vi "RS-xxx Factory.vi"(8 "error in (no error)":errorcluster, 10 "RS-xxx settings":T1) -> (0 "error out":errorcluster, 3 "RS-xxx out":refnum<class "RS-xxx.lvclass">)   [LabVIEW 2018, in "Protocols.lvlib" / "RS-xxx.lvclass"]
doc: "Instantiate an RS-xxx Protocol Object using the provided RS-xxx Port Settings\n\nInput: \nPort: specifies the resource to be opened.\nBaud Rate: is the rate of transmission.\nData Bits: is the number of bits in the incoming data.The value of data bits is between five and eight.\nParity: specifies the parity used for every frame to be transmitted or received. This input accepts the following values. \n\n 0 - no parity (default) \n 1 - odd parity \n 2 - even parity \n 3 - mark parity \n 4 - space parity\n\nFlow Control: sets the type of control used by the transfer mechanism. This input accepts the following values.\n\n 0 - None (default)—The transfer mechanism does not use flow control. Buffers on both sides of the connection are assumed to be large enough to hold all data transferred. \n 1 - XON/XOFF—The transfer mechanism uses the XON and XOFF characters to perform flow control. The transfer mechanism controls input flow by sending XOFF when the receive buffer is nearly full, and it controls the output flow by suspending transmission when XOFF is received. \n 2 - RTS/CTS—The transfer mechanism uses the RTS output signal and the CTS input signal to perform flow control. The transfer mechanism controls input flow by unasserting the RTS signal when the receive buffer is nearly full, and it controls output flow by suspending the transmission when the CTS signal is unasserted. \n 3 - XON/XOFF and RTS/CTS—The transfer mechanism uses the XON and XOFF characters and the RTS output signal and CTS input signal to perform flow control. The transfer mechanism controls input flow by sending XOFF and unasserting the RTS signal when the receive buffer is nearly full, and it controls the output flow by suspending transmission when XOFF is received and the CTS is unasserted. \n 4 - DTR/DSR—The transfer mechanism uses the DTR output signal and the DSR input signal to perform flow control. The transfer mechanism controls input flow by unasserting the DTR signal when the receive buffer is nearly full, and it controls output flow by suspending the transmission when the DSR signal is unasserted. \n 5 - XON/XOFF and DTR/DSR—The transfer mechanism uses the XON and XOFF characters and the DTR output signal and DSR input signal to perform flow control. The transfer mechanism controls input flow by sending XOFF and unasserting the DTR signal when the receive buffer is nearly full, and it controls the output flow by suspending transmission when XOFF is received and the DSR signal is unasserted. \n\nXON: specifies the XON character\nXOFF: specifies the XOFF character\nEnd Read on Termination Character: ends reading the transfered data when encountering the specified termination character\nEnd Write on Termination Character: ends writing the message when encountering the specified termination character\n\nOutput:\n\nRS-xxx Out: RS-xxx object created using the provided RS-xxx Settings"
uses:
  RS-xxx.lvclass
  RS-xxx Settings.ctl
  RS-xxx.lvclass/RS-xxx.ctl
  Data Access/Write PortSettings.vi
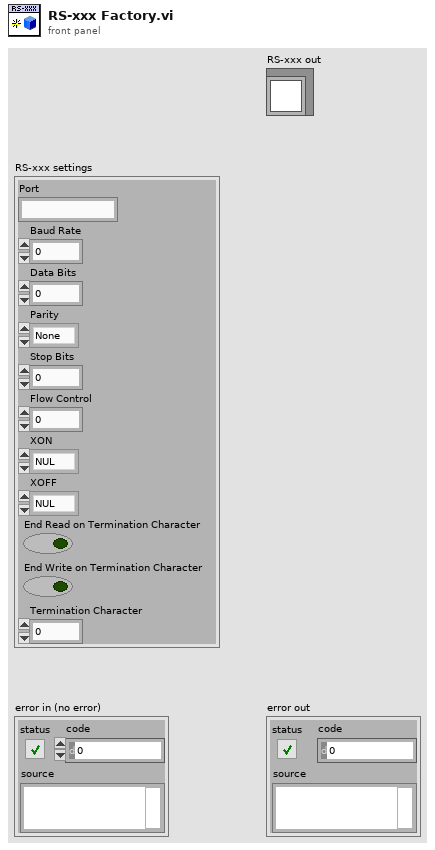
[diagram p1: front panel]
types:
  T1 = typedef "Protocols.lvlib/RS-xxx.lvclass/RS-xxx Settings.ctl" = cluster{"Port":string, "Baud Rate":u32, "Data Bits":u16, "Parity":enum16{"None", "Odd", "Even", "Mark", "Space"}, "Stop Bits":u16, "Flow Control":u16, "XON":enum16{"NUL", "SOH", "STX", "ETX", "EOT", "ENQ", "ACK", "BEL", "BS", "HT", "LF", "VT", "FF", "CR", "SO", "SI", "DLE", "DC1", "DC2", "DC3", "DC4", "NAK", "SYN", "ETB", "CAN", "EM", "SUB", "ESC", "FS", "GS", "RS", "US", "SP", "!", "\"", "#", "$", "%", "&", "'", "(", ")", "*", "+", ",", "- (-)", ".", "/", "0", "1", "2", "3", "4", "5", "6", "7", "8", "9", ":", ";", "<", "=", ">", "?", "@", "A", "B", "C", "D", "E", "F", "G", "H", "I", "J", "K", "L", "M", "N", "O", "P", "Q", "R", "S", "T", "U", "V", "W", "X", "Y", "Z", "[", "\\", "]", "^", "_", "`", "a", "b", "c", "d", "e", "f", "g", "h", "i", "j", "k", "l", "m", "n", "o", "p", "q", "r", "s", "t", "u", "v", "w", "x", "y", "z", "{", "|", "}", "~"}, "XOFF":enum16{"NUL", "SOH", "STX", "ETX", "EOT", "ENQ", "ACK", "BEL", "BS", "HT", "LF", "VT", "FF", "CR", "SO", "SI", "DLE", "DC1", "DC2", "DC3", "DC4", "NAK", "SYN", "ETB", "CAN", "EM", "SUB", "ESC", "FS", "GS", "RS", "US", "SP", "!", "\"", "#", "$", "%", "&", "'", "(", ")", "*", "+", ",", "- (-)", ".", "/", "0", "1", "2", "3", "4", "5", "6", "7", "8", "9", ":", ";", "<", "=", ">", "?", "@", "A", "B", "C", "D", "E", "F", "G", "H", "I", "J", "K", "L", "M", "N", "O", "P", "Q", "R", "S", "T", "U", "V", "W", "X", "Y", "Z", "[", "\\", "]", "^", "_", "`", "a", "b", "c", "d", "e", "f", "g", "h", "i", "j", "k", "l", "m", "n", "o", "p", "q", "r", "s", "t", "u", "v", "w", "x", "y", "z", "{", "|", "}", "~"}, "End Read on Termination Character":bool, "End Write on Termination Character":bool, "Termination Character":u8}
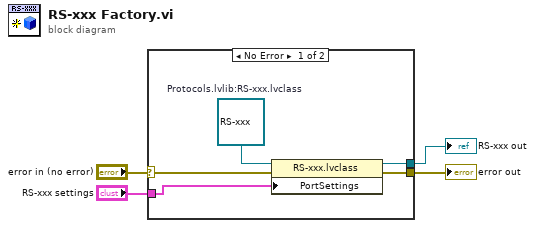
[diagram p0: block diagram]
diagram:
  n1 = case shown="No Error" "error in (no error)" {
    selector: "error in (no error)" -> [w5 w10]
    tunnel: "RS-xxx settings" -> [w8 _]
    tunnel: [w7 _] -> w3
    tunnel: [w6 w10] -> w2
    frame No Error {
      w9 = refnum<class "RS-xxx.lvclass"> refnum  # Protocols.lvlib:RS-xxx.lvclass
      n2 = property class="RS-xxx.lvclass"(reference=w9, error in=w5, "PortSettings"=w8) -> (reference out=w7:refnum<class "RS-xxx.lvclass">, error out=w6:errorcluster)
    }
    frame Error {
    }
  }
  "RS-xxx out" <- w3
  "error out" <- w2
